vi "WSVCAP SHL FPGA LL I2C Read Data.vi"(11 "error in (no error)":errorcluster, 12 "UUT Set (0-1) (Legacy)":u8, 13 "Socket Mask":u64 format="%012x") -> (4 "Long Word Out (1-Bit for Each Channel)":u64, 15 "error out":errorcluster)   [LabVIEW 2017]
uses:
  <vilib>/rvi/eio/common/nirviEmuTemplateMethod_errors.vi
  <vilib>/eio/EIONode/EIONode.xnode
  WSVCAP SHL FPGA LL I2C Debug Global.vi
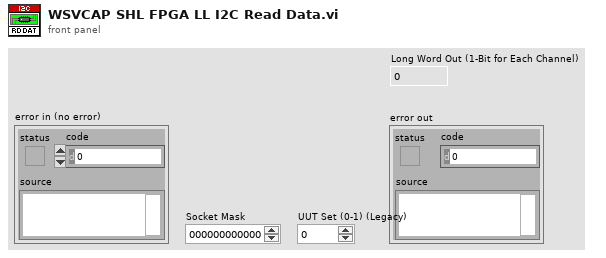
[diagram p1: front panel]
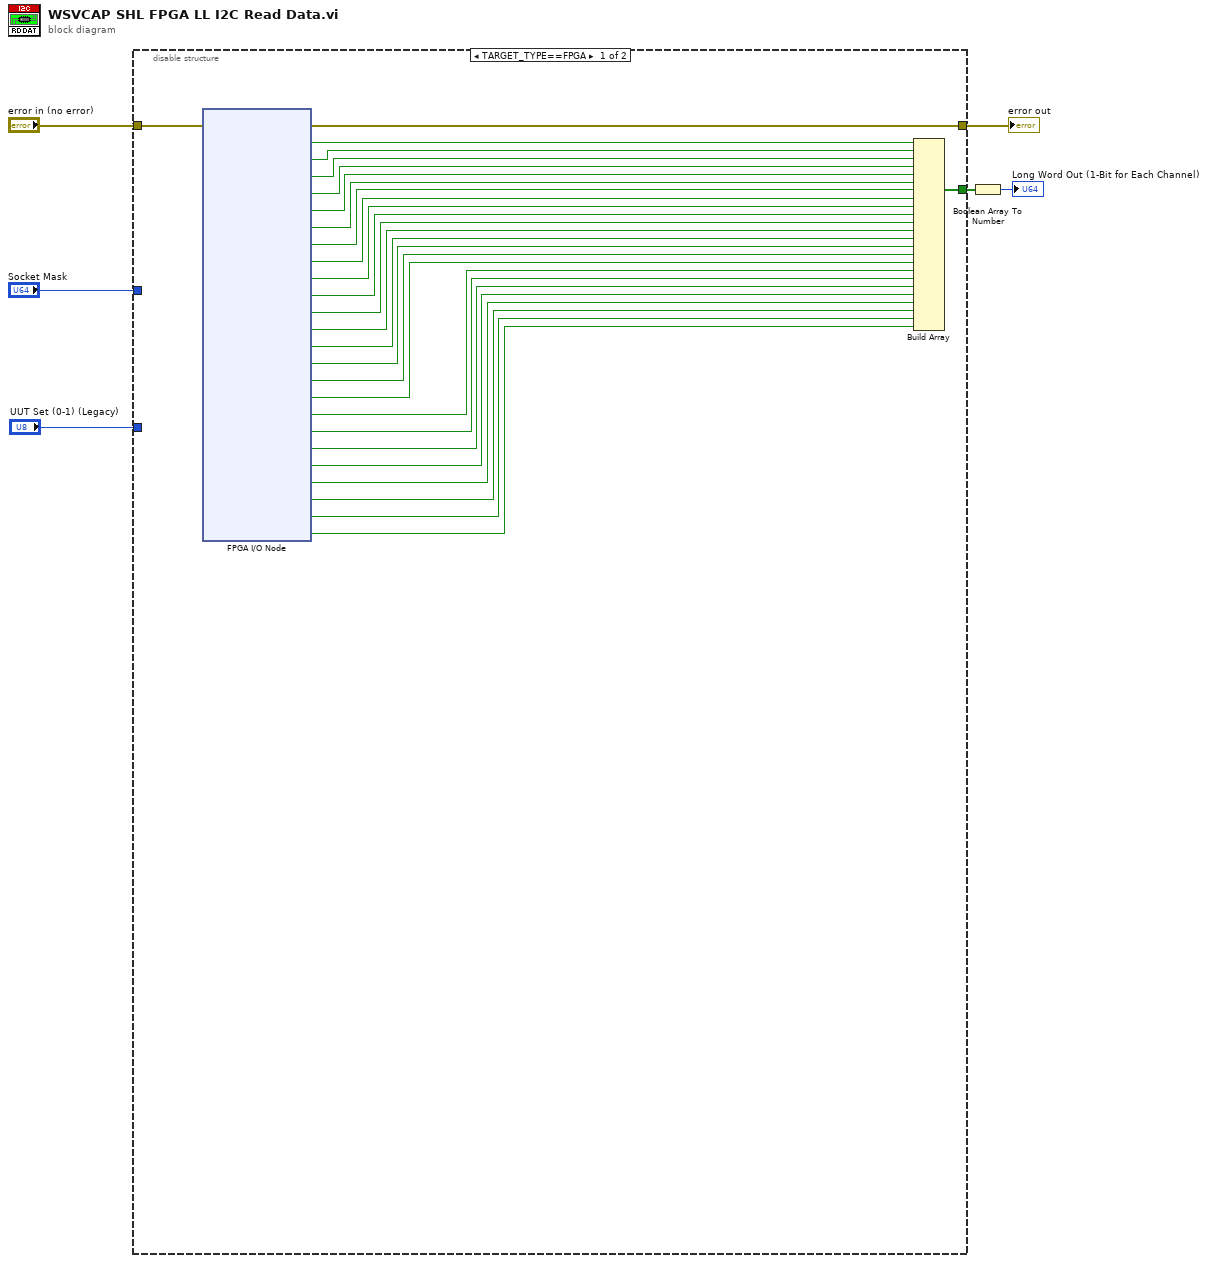
[diagram p0: block diagram]
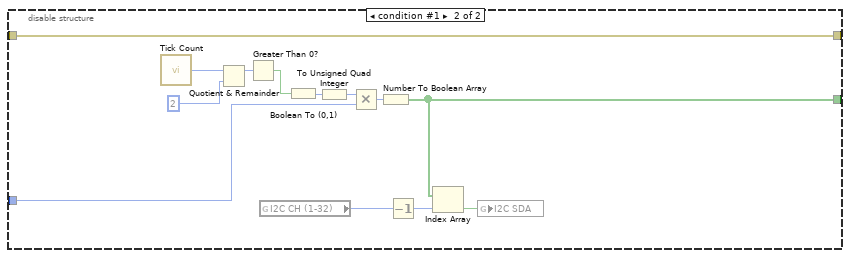
[diagram p2: hidden frame]
diagram:
  n1 = disable-structure shown="TARGET_TYPE==FPGA" {
    disable-tunnel: [w33 w43] -> w6
    disable-tunnel: "error in (no error)" -> [w32 w43]
    disable-tunnel: "Socket Mask" -> [_ w40]
    disable-tunnel: [w9 w34] -> w2
    disable-tunnel: "UUT Set (0-1) (Legacy)" -> [_ _]
    frame condition #0 (active) {
      n2 = xnode "FPGA I/O Node"("error in"=w32) -> ("error out"=w33:errorcluster, "I2C_SDA_S1"=w31:bool, "I2C_SDA_S2"=w30:bool, "I2C_SDA_S3"=w29:bool, "I2C_SDA_S4"=w28:bool, "I2C_SDA_S5"=w27:bool, "I2C_SDA_S6"=w26:bool, "I2C_SDA_S7"=w25:bool, "I2C_SDA_S8"=w24:bool, "I2C_SDA_S9"=w23:bool, "I2C_SDA_S10"=w22:bool, "I2C_SDA_S11"=w21:bool, "I2C_SDA_S12"=w20:bool, "I2C_SDA_S13"=w19:bool, "I2C_SDA_S14"=w18:bool, "I2C_SDA_S15"=w17:bool, "I2C_SDA_S16"=w8:bool, "I2C_SDA_S17"=w7:bool, "I2C_SDA_S18"=w16:bool, "I2C_SDA_S19"=w15:bool, "I2C_SDA_S20"=w14:bool, "I2C_SDA_S21"=w13:bool, "I2C_SDA_S22"=w12:bool, "I2C_SDA_S23"=w11:bool, "I2C_SDA_S24"=w10:bool)  [unwired: 24 in, 24 out]
      n3 = Build Array(w31, w30, w29, w28, w27, w26, w25, w24, w23, w22, w21, w20, w19, w18, w17, w8, w7, w16, w15, w14, w13, w12, w11, w10) -> (w9:bool[])
    }
    frame condition #1 {
      n4 = call "Tick Count"() -> ("Tick Count(Ticks)"=w46:u32)
      n5 = Quotient & Remainder(x=w46, y=u32 2) -> (x-y*floor(x/y)=w45:u32)  [unwired: 1 out]
      n6 = Greater Than 0?(x=w45) -> (x > 0?=w42:bool)
      n7 = global read "WSVCAP SHL FPGA LL I2C Debug Global.vi" "I2C CH (1-32)"() -> (w39:i32)
      n8 = Boolean To (0,1)(Boolean=w42) -> (0, 1=w41:i16)
      n9 = To Unsigned Quad Integer(1:w41) -> (0:w38:u64)
      n10 = Multiply(x=w38, y=w40) -> (x*y=w37:u64)
      n11 = Number To Boolean Array(number=w37) -> (Boolean array=w34:bool[])
      n12 = Decrement(x=w39) -> (x-1=w35:i32)
      n13 = Index Array(array=w34, index=w35) -> (element=w36:bool)
      n14 = global write "WSVCAP SHL FPGA LL I2C Debug Global.vi" "I2C SDA"(w36) -> ()
    }
  }
  "error out" <- w6
  n15 = Boolean Array To Number(Boolean array=w2) -> (number=→"Long Word Out (1-Bit for Each Channel)":u64)
